vi "Sett_UP_Convert.vi"(8 "error in (no error)":errorcluster, 9 "Divider(1)":dbl=1.0, 11 "ISO 14443 B UP in":refnum<class "ISO 14443 B UP.lvclass">) -> (0 "error out":errorcluster, 2 "Waveform":waveform(dbl), 3 "ISO 14443 B UP out":refnum<class "ISO 14443 B UP.lvclass">)   [LabVIEW 2019, in "ISO 14443 B UP.lvclass"]
uses:
  ISO 14443 B UP.lvclass
  ISO 14443 B UP.lvclass/ISO 14443 B UP.ctl
  <vilib>/addons/Modulation/Analog/support/mod_Set Error Source.vi
  <vilib>/addons/Modulation/Digital/Support/Common/Validators/mod_Generate Filter Coefficients Validate.vi
  <vilib>/addons/Modulation/Digital/General/subVIs/mod_Generate Filter Coefficients.vi
  <vilib>/addons/Modulation/Digital/General/MT Generate ASK system parameters (M).vi
  <vilib>/addons/Modulation/niDMT.lvlib
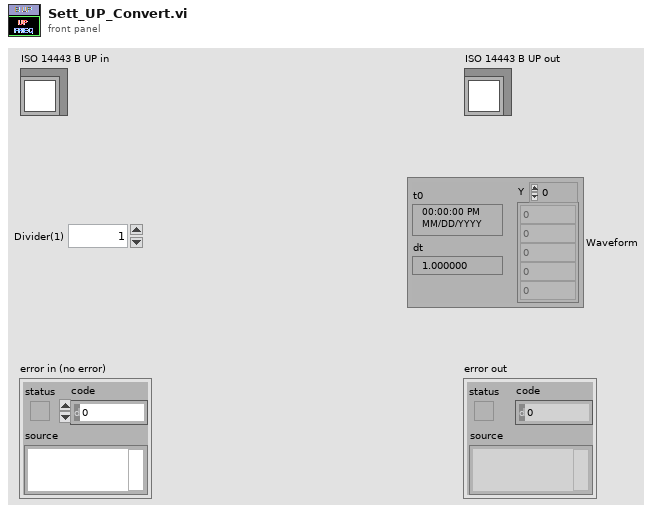
[diagram p1: front panel]
types:
  T1 = enum16{"none", "Raised Cosine", "Root Raised Cos", "Gaussian"}
  T2 = enum16{"FSK", "PSK", "QAM", "MSK", "PAM", "ASK", "CPM"}
  T3 = cluster{"samples per symbol (16)":i32, "symbol map":cdb[]}
  T4 = typedef "niAMT.lvlib/Complex Data Waveform.ctl" = cluster{"t0":dbl, "dt":dbl, "Y":cdb[]}
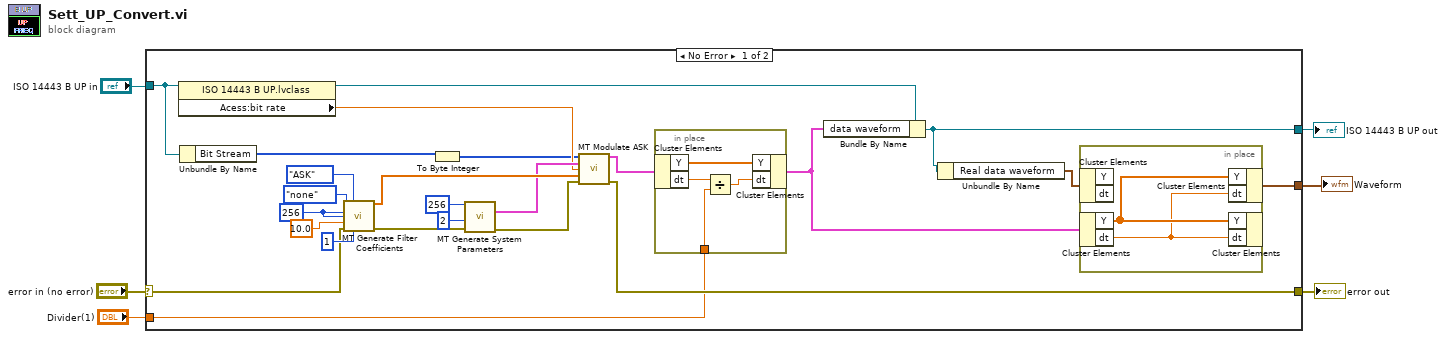
[diagram p0: block diagram]
diagram:
  n1 = case shown="No Error" "error in (no error)" {
    selector: "error in (no error)" -> [w17 w37]
    tunnel: [w15 w37] -> w3
    tunnel: "ISO 14443 B UP in" -> [w30 w38]
    tunnel: [w10 w38] -> w2
    tunnel: [w7 _] -> w1
    tunnel: "Divider(1)" -> [w14 _]
    frame No Error {
      w25 = 256 ("pulse shaping samples per symbol (16)")
      n2 = property class="ISO 14443 B UP.lvclass"(reference=w30) -> (reference out=w16:refnum<class "ISO 14443 B UP.lvclass">, "Acess:bit rate"=w18:dbl)  [unwired: 1 in, 1 out]
      n3 = Unbundle By Name(w30) -> ("Bit Stream"=w13:u8[])
      n4 = call <vilib>:"MT Generate Filter Coefficients.vi"("pulse shaping filter (none)"=T1."none", "modulation type"=T2."ASK", "pulse shaping samples per symbol (16)"=w25, "matched samples per symbol (16)"=w25, "filter parameter"=10.0, "error in (no error)"=w17, "filter length (symbols)"=1) -> ("pulse shaping filter coefficients"=w27:dbl[], "error out"=w22:errorcluster)  [unwired: 7 out]
      n5 = To Byte Integer(number=w13) -> (8bit integer=w12:i8[])
      n6 = call-poly <vilib>:"MT Generate System Parameters.vi"("samples per symbol (16)"=256, "M-ASK (2)"=2, "error in (no error)"=w22) -> ("ASK system parameters"=w19:T3, "error out"=w20:errorcluster)  [unwired: 11 out]
      n7 = call <vilib>:"MT Modulate ASK.vi"("input bit stream"=w12, "ASK system parameters"=w19, "symbol rate (Hz)"=w18, "pulse shaping filter coefficients"=w27, "error in (no error)"=w20) -> ("output complex waveform"=w11:T4, "error out"=w15:errorcluster)  [unwired: 8 in, 1 out]
      n8 = in-place {
        in-place-border: w14 -> [w36]
        n9 = in-place-cluster #1(w11) -> ("Y"=w33:cdb[], "dt"=w35:dbl)
        n10 = Divide(x=w35, y=w36) -> (x/y=w34:dbl)
        n11 = in-place-cluster #1("Y"=w33, "dt"=w34) -> (w8:T4)
      }
      n12 = Bundle By Name(cluster=w16, "data waveform"=w8) -> (w10:refnum<class "ISO 14443 B UP.lvclass">)
      n13 = Unbundle By Name(w10) -> ("Real data waveform"=w9:waveform(dbl))
      n14 = in-place {
        n15 = in-place-cluster #2(w9) -> ()  [unwired: 2 out]
        n16 = in-place-cluster #3(w8) -> ("Y"=w32:cdb[], "dt"=w31:dbl)
        n17 = in-place-cluster #2("Y"=w32, "dt"=w31) -> (w7:waveform(dbl))
        n18 = in-place-cluster #3("Y"=w32, "dt"=w31) -> ()  [unwired: 1 out]
      }
    }
    frame Error {
    }
  }
  "error out" <- w3
  "ISO 14443 B UP out" <- w2
  "Waveform" <- w1
